vi "gyro-pll-V2.vi"() -> ()   [LabVIEW 2017]
uses:
  lorentzian.ctl
  circle corners.ctl
  pid -- parameters.ctl
  <vilib>/event_ctls.llb/eventvkey.ctl
  cursor winow.ctl
  show-win- control.ctl
  PID action.ctl
  PLL data source.ctl
  cursor window action.ctl
  agregator -- action.ctl
  interpolation state - real.ctl
  data source action.ctl
  four-corner circle transformation.ctl
  cursor action.ctl
  publisher action.ctl
  d67dc248-e042-8a4a-b341-023c3e33f963.vi
  linear interpolation - real.vi
  <vilib>/Array/Sort 2D Array - Pop Stack.vi
  <vilib>/Array/Sort 2D Array - Push Stack.vi
  draw a line.vi
  draw a circle.vi
  linear interpolation iiii- complex.vi
  Q - not nan -- real.vi
  generate linear region.vi
panel:
  in  "all 3":enum32{"all", "other"}(tab)
  in  "reset freq! :r":bool
  in  "dt (sec)":dbl=0.05 format="%#_10f"
  out "Plot: complex plane - filter":cluster{dbl[], dbl[]}[](graph)=[{[1.2813614834440607e-05, 1.2784806307815229e-05, 1.2698431267884004e-05, 1.2554641245817403e-05, 1.235368849817431e-05, 1.2095925564358299e-05, 1.17818046481437e-05, 1.1411876824356577e-05, 1.0986791072102168e-05, 1.0507293136235029e-05, 9.97422421906916e-06, 9.388519504623323e-06, 8.75120651799044e-06, 8.063403322709483e-06, 7.326316559302067e-06, 6.54123932841497e-06, 5.709548922282207e-06, 4.832704408486439e-06, 3.912244070258618e-06, 2.949782707806539e-06, 1.947008805406491e-06, 9.056815692281653e-07, -1.7237215891082665e-07, -1.2852611064461961e-06, -2.431032888001771e-06, -3.6076774305368316e-06, -4.81313049969727e-06, -6.045277321184067e-06, -7.301956290786042e-06, -8.580962766568125e-06, -9.880052936562472e-06, -1.1196947755177101e-05, -1.2529336941416313e-05, -1.3874883031898544e-05, -1.5231225481561452e-05, -1.6595984804860076e-05, -1.7966766750193015e-05, -1.9341166500233316e-05, -2.0716772890795228e-05, -2.209117264083553e-05, -2.3461954586168464e-05, -2.4826713909467085e-05, -2.618305635913e-05, -2.752860244961223e-05, -2.886099163585144e-05, -3.017788645446607e-05, -3.147697662446042e-05, -3.2755983100242503e-05, -3.401266206984447e-05, -3.524480889133127e-05, -3.6450261960491715e-05, -3.762690650302677e-05, -3.877267828458235e-05, -3.9885567232117724e-05, -4.0963620960256705e-05, -4.200494819643504e-05, -4.300772209883508e-05, -4.3970183461287165e-05, -4.4890643799514986e-05, -4.576748831331076e-05, -4.659917871944352e-05, -4.738425595033061e-05, -4.8121342713738026e-05, -4.8809145909018984e-05, -4.9446458895651866e-05, -5.003216361009771e-05, -5.056523252726357e-05, -5.104473046313072e-05, -5.1469816215385134e-05, -5.183974403917225e-05, -5.215386495538684e-05, -5.241162788920287e-05, -5.2612580636845954e-05, -5.275637065891256e-05, -5.2842745698843786e-05, -5.2871554225469164e-05, -5.2842745698843786e-05, -5.275637065891256e-05, -5.2612580636845954e-05, -5.241162788920287e-05, -5.2153864955386856e-05, -5.183974403917226e-05, -5.1469816215385134e-05, -5.104473046313072e-05, -5.0565232527263586e-05, -5.003216361009772e-05, -4.944645889565188e-05, -4.8809145909019e-05, -4.812134271373804e-05, -4.738425595033063e-05, -4.659917871944353e-05, -4.576748831331078e-05, -4.4890643799515e-05, -4.397018346128718e-05, -4.3007722098835096e-05, -4.200494819643505e-05, -4.096362096025673e-05, -3.9885567232117744e-05, -3.8772678284582364e-05, -3.762690650302679e-05, -3.645026196049173e-05, -3.5244808891331293e-05, -3.401266206984449e-05, -3.275598310024252e-05, -3.1476976624460435e-05, -3.0177886454466085e-05, -2.8860991635851447e-05, -2.7528602449612266e-05, -2.6183056359130033e-05, -2.4826713909467122e-05, -2.3461954586168495e-05, -2.209117264083556e-05, -2.0716772890795258e-05, -1.9341166500233336e-05, -1.796676675019304e-05, -1.65959848048601e-05, -1.5231225481561472e-05, -1.387488303189856e-05, -1.2529336941416328e-05, -1.1196947755177116e-05, -9.880052936562479e-06, -8.580962766568159e-06, -7.301956290786074e-06, -6.045277321184099e-06, -4.813130499697297e-06, -3.6076774305368553e-06, -2.431032888001795e-06, -1.2852611064462199e-06, -1.7237215891084359e-07, 9.056815692281483e-07, 1.9470088054064774e-06, 2.949782707806522e-06, 3.912244070258608e-06, 4.832704408486426e-06, 5.7095489222822e-06, 6.541239328414966e-06, 7.3263165593020436e-06, 8.063403322709466e-06, 8.751206517990427e-06, 9.388519504623309e-06, 9.97422421906915e-06, 1.0507293136235015e-05, 1.0986791072102155e-05, 1.1411876824356577e-05, 1.17818046481437e-05, 1.2095925564358292e-05, 1.235368849817431e-05, 1.2554641245817403e-05, 1.2698431267884004e-05, 1.2784806307815229e-05], [3.545285490891632e-05, 3.682815960626468e-05, 3.820105155184222e-05, 3.956912222666456e-05, 4.0929971569894545e-05, 4.2281212189364424e-05, 4.3620473549873006e-05, 4.4945406131909886e-05, 4.625368555351105e-05, 4.754301664801469e-05, 4.881113749056338e-05, 5.0055823366288934e-05, 5.127489067321824e-05, 5.246620075305308e-05, 5.362766364310354e-05, 5.4757241742792726e-05, 5.585295338830057e-05, 5.6912876329075535e-05, 5.7935151100115256e-05, 5.891798428410004e-05, 5.9859651657656206e-05, 6.0758501216229826e-05, 6.161295607226402e-05, 6.24215172215956e-05, 6.31827661732177e-05, 6.389536743779506e-05, 6.455807087056606e-05, 6.516971386452149e-05, 6.572922339001227e-05, 6.623561787720805e-05, 6.668800893810432e-05, 6.708560292505672e-05, 6.742770232310883e-05, 6.771370697367026e-05, 6.794311512739893e-05, 6.811552432443979e-05, 6.823063210047616e-05, 6.8288236517355e-05, 6.8288236517355e-05, 6.823063210047616e-05, 6.811552432443979e-05, 6.794311512739893e-05, 6.771370697367026e-05, 6.742770232310883e-05, 6.708560292505674e-05, 6.668800893810432e-05, 6.623561787720805e-05, 6.572922339001227e-05, 6.516971386452149e-05, 6.455807087056606e-05, 6.389536743779506e-05, 6.31827661732177e-05, 6.242151722159561e-05, 6.161295607226403e-05, 6.075850121622983e-05, 5.985965165765622e-05, 5.8917984284100045e-05, 5.793515110011527e-05, 5.691287632907554e-05, 5.585295338830058e-05, 5.475724174279273e-05, 5.362766364310355e-05, 5.246620075305309e-05, 5.1274890673218255e-05, 5.005582336628895e-05, 4.8811137490563386e-05, 4.7543016648014695e-05, 4.625368555351106e-05, 4.4945406131909906e-05, 4.3620473549873027e-05, 4.228121218936444e-05, 4.092997156989456e-05, 3.9569122226664574e-05, 3.8201051551842225e-05, 3.682815960626469e-05, 3.545285490891634e-05, 3.407755021156798e-05, 3.270465826599045e-05, 3.13365875911681e-05, 2.9975738247938106e-05, 2.8624497628468227e-05, 2.7285236267959645e-05, 2.596030368592278e-05, 2.4652024264321608e-05, 2.336269316981797e-05, 2.209457232726928e-05, 2.0849886451543717e-05, 1.963081914461441e-05, 1.8439509064779572e-05, 1.727804617472912e-05, 1.614846807503993e-05, 1.5052756429532084e-05, 1.3992833488757123e-05, 1.2970558717717392e-05, 1.198772553373261e-05, 1.1046058160176439e-05, 1.0147208601602828e-05, 9.292753745568634e-06, 8.484192596237056e-06, 7.72294364461495e-06, 7.010342380037596e-06, 6.347638947266588e-06, 5.735995953311157e-06, 5.176486427820386e-06, 4.670091940624589e-06, 4.2177008797283295e-06, 3.820106892775922e-06, 3.478007494723825e-06, 3.1920028441623845e-06, 2.9625946904337074e-06, 2.7901854933928613e-06, 2.675077717356487e-06, 2.6174733004776394e-06, 2.6174733004776394e-06, 2.675077717356487e-06, 2.7901854933928545e-06, 2.9625946904337074e-06, 3.1920028441623777e-06, 3.4780074947238183e-06, 3.820106892775915e-06, 4.217700879728323e-06, 4.670091940624575e-06, 5.176486427820369e-06, 5.7359959533111404e-06, 6.347638947266571e-06, 7.010342380037572e-06, 7.722943644614927e-06, 8.484192596237036e-06, 9.292753745568607e-06, 1.0147208601602805e-05, 1.1046058160176422e-05, 1.1987725533732593e-05, 1.2970558717717375e-05, 1.3992833488757099e-05, 1.5052756429532063e-05, 1.6148468075039908e-05, 1.7278046174729072e-05, 1.8439509064779535e-05, 1.9630819144614373e-05, 2.084988645154368e-05, 2.209457232726924e-05, 2.3362693169817932e-05, 2.465202426432157e-05, 2.5960303685922738e-05, 2.7285236267959618e-05, 2.86244976284682e-05, 2.9975738247938083e-05, 3.133658759116807e-05, 3.270465826599042e-05, 3.407755021156795e-05]}, {[-4.107222204249114e-06, -5.699396953375631e-06, -7.291571702502146e-06, -8.883746451628662e-06, -1.0475921200755179e-05, -1.2068095949881695e-05, -1.366027069900821e-05, -1.5252445448134727e-05, -1.6844620197261244e-05, -1.843679494638776e-05, -2.0028969695514277e-05, -2.1621144444640793e-05, -2.3213319193767307e-05, -2.4805493942893823e-05, -2.639766869202034e-05, -2.7989843441146856e-05, -2.9582018190273373e-05, -3.1174192939399886e-05, -3.2766367688526406e-05, -3.4358542437652926e-05], [6.727721046188663e-06, 9.60023443246143e-06, 1.2472747818734195e-05, 1.534526120500696e-05, 1.8217774591279727e-05, 2.1090287977552493e-05, 2.396280136382526e-05, 2.6835314750098024e-05, 2.970782813637079e-05, 3.2580341522643556e-05, 3.545285490891632e-05, 3.832536829518909e-05, 4.1197881681461854e-05, 4.407039506773462e-05, 4.6942908454007386e-05, 4.981542184028015e-05, 5.268793522655292e-05, 5.556044861282568e-05, 5.843296199909845e-05, 6.130547538537121e-05]}, {[-4.875410355824193e-05, -4.5881590171969166e-05, -4.30090767856964e-05, -4.0136563399423635e-05, -3.726405001315087e-05, -3.43915366268781e-05, -3.1519023240605344e-05, -2.8646509854332574e-05, -2.577399646805981e-05, -2.2901483081787043e-05, -2.0028969695514277e-05, -1.7156456309241514e-05, -1.4283942922968748e-05, -1.1411429536695983e-05, -8.538916150423217e-06, -5.666402764150451e-06, -2.793889377877685e-06, 7.862400839508097e-08, 2.951137394667847e-06, 5.823650780940613e-06], [1.953110741765116e-05, 2.1123282166777676e-05, 2.2715456915904193e-05, 2.430763166503071e-05, 2.5899806414157222e-05, 2.7491981163283742e-05, 2.9084155912410256e-05, 3.067633066153677e-05, 3.226850541066329e-05, 3.386068015978981e-05, 3.545285490891632e-05, 3.7045029658042835e-05, 3.863720440716935e-05, 4.022937915629587e-05, 4.182155390542239e-05, 4.34137286545489e-05, 4.5005903403675415e-05, 4.6598078152801935e-05, 4.8190252901928455e-05, 4.978242765105497e-05]}, {[-6.155748992970442e-05, -5.581246315715889e-05, -5.006743638461336e-05, -4.432240961206783e-05, -3.85773828395223e-05, -3.2832356066976766e-05, -2.7087329294431234e-05, -2.1342302521885702e-05, -1.559727574934017e-05, -9.852248976794639e-06, -4.107222204249107e-06, 1.6378045682964245e-06, 7.382831340841956e-06, 1.3127858113387488e-05, 1.887288488593302e-05, 2.461791165847855e-05, 3.0362938431024083e-05, 3.6107965203569615e-05, 4.185299197611515e-05, 4.759801874866068e-05], [-2.5115773936341655e-05, -2.1931424438088622e-05, -1.874707493983559e-05, -1.556272544158256e-05, -1.2378375943329526e-05, -9.194026445076493e-06, -6.009676946823463e-06, -2.8253274485704296e-06, 3.5902204968260365e-07, 3.543371547935637e-06, 6.72772104618867e-06, 9.912070544441703e-06, 1.309642004269473e-05, 1.6280769540947763e-05, 1.9465119039200796e-05, 2.264946853745383e-05, 2.5833818035706863e-05, 2.9018167533959896e-05, 3.220251703221293e-05, 3.538686653046596e-05]}]
  in  "PID parameters :{}[]":T1={"I (sec)"=1.05568883726763, "P (sec)"=1.0091249923988408} {"P (sec)" scale=0.01..10.0; "I (sec)" scale=0.01..10.0}
  in  "visc hist time (sec)":dbl=5.0 format="%#_10f"
  in  "circle lorentzian":T2={"Amplitude (V)"=0.0014148170690314607, "omega0 (Hz)"=45421.57991847975, "Gamma (Hz)"=43.078737233394115, "phase (rad)"=3.647715388411055, "Q"=1054.3851290810235, "Norm  Ampl"=nan, "z (inf)"=-4.107222204249114e-06+6.727721046188663e-06i, "4corners"={"z (-pi/2)"=-4.875410355824193e-05+1.9531107417651163e-05i, "z(inf)"=-4.107222204249114e-06+6.727721046188663e-06i, "z (pi/2)"=8.696164167213385e-06+5.137460240018148e-05i, "z center"=-2.0028969695514273e-05+3.545285490891632e-05i, "z(0)"=-3.595071718677943e-05+6.417798877164398e-05i, "radius"=3.2842584529954884e-05}} {"z (inf)" format="%#9_9f"; "Q" format="%#9_9f"; "phase (rad)" format="%#9_9f"; "Gamma (Hz)" format="%#9_9f"; "omega0 (Hz)" format="%#9_9f"}
  in  "time int ave time (sec)":dbl=0.05 format="%#_10f"
  in  "get fit! :q":bool
  in  "PLL away! :@":bool
  out "zi freq (Hz)":dbl=45590.53325451146 format="%#.4f"
  out "delta freq (Hz)":dbl=168.9533360317073 format="%#.8f"
  in  "PLL limits (Hz)":dbl=5000.0 format="%#.2f"
  in  "PLL data source":T4=enum."MFLI"
  in  "cursor bracket: fit boundaries":T5={"left"=20223.692861806387, "right "=24717.846831096696, "center"=22470.76984645154, "window"=4494.153969290309, "cursors"=[0, 1, 2], "relative"=0, "absolute"=0, "fixed vertical offset"=0.0, "vertical offset"=0.0, "skew"=0.0, "default window frac"=0.1, "kind"=enum."symmetric", "skew.left"=0.5, "skew.right"=0.5, "Plot ref"=refnum, "wing order"=enum."forw"}
  out "VKey":T6
  out "Char":i16=122
  in  "lorentzian -- basic":T2={"Amplitude (V)"=1.0, "omega0 (Hz)"=1000.0, "Gamma (Hz)"=3.0, "phase (rad)"=0.0, "Q"=300.0, "Norm  Ampl"=nan, "z (inf)"=0.0+0.0i, "4corners"={"z (-pi/2)"=9.277908004825974e-07+0.0007240755403629966i, "z(inf)"=2.6527949823343002e-05+0.0007477540585896028i, "z (pi/2)"=2.8494315967368497e-06+0.0007733542176124632i, "z center"=1.8886111986097237e-06+0.0007487148789877299i, "z(0)"=-2.2750727426123552e-05+0.000749675699385857i, "radius"=2.4658065287076567e-05}} {"z (inf)" format="%#9_9f"; "Q" format="%#9_9f"; "phase (rad)" format="%#9_9f"; "Gamma (Hz)" format="%#9_9f"; "omega0 (Hz)" format="%#9_9f"}
  out "DO reset freq !":bool
  in  "save lor for later":bool
  in  "reset lorentzian from basic":bool
  in  "Do reset frequency source":dbl=15.0 format="%#_10f"
  in  "Do reset frequency -- PID action":T7=enum."reset frequency"
  in  "all":enum32{"all", "other"}(tab)
  in  "reset win from freq !":bool
  in  "reset freq from win !":bool
  in  "send for fit!":bool
  out "Plot: complex- hist":cluster{dbl[], dbl[]}[](graph)=[{[-1.281770488197954e-05, -1.0986465994251437e-05, -6.882277068596139e-06, -1.0956775876071293e-05, -6.698135551181071e-06, -4.290132536004875e-06, -9.884114205234754e-06, -1.0020825799021037e-05, -1.0594885594792778e-05, -1.1315291508425677e-05, -9.15588407390866e-06, -4.631085114607762e-06, -9.91714593188108e-06, -1.1229612675301296e-05, -3.7616560713859013e-06, -8.359687227641351e-06, -1.2250832382384907e-05, -7.790134627243845e-06, -9.342526339103081e-06, -1.4326621095772142e-05, -1.5233280532867308e-05, -8.680230516053846e-06, -1.0092209301965068e-05, -1.1126455180992973e-05, -1.450326589164611e-05, -5.246423985745027e-06, -3.6636994414210996e-06, -5.141838176586089e-06, -1.0012731994795598e-05, -1.5335458675967136e-05, -1.5049525631563538e-05, -1.6069153025824554e-05, -8.141448343003425e-06, -7.412163963946879e-06, -1.2430596668377613e-05, -1.3231583279096937e-05, -6.985101526890639e-06, -6.490446532337178e-06, -9.373512369438486e-06, -1.2126573717328789e-05, -1.589980051855066e-05, -1.1354584338626872e-05, -8.824369474721001e-06, -9.99549965874622e-07, -6.288455267304482e-06, -7.484835846038533e-06, -1.351758082676016e-05, -9.828075336477092e-06, -1.1524401297069373e-05, -1.587464391008797e-05, -1.0557451032928354e-05, -1.3139806431129755e-05, -1.2011711561005575e-05, -1.1843224223572645e-05, -1.37278337116776e-05, -1.6522056027489975e-05, -1.2383234897091292e-05, -8.10061086687687e-06, -5.225988471535249e-06, -3.4747132306206463e-06, -9.256075255275086e-06, -1.113538910524981e-05, -1.0058288945367669e-05, -1.0233727177421544e-05, -8.648566858261817e-06, -8.711623226434552e-06, -1.1066342002860999e-05, -1.1269186189822962e-05, -9.535872752272664e-06, -7.947195421785513e-06, -2.452968790242578e-06, -8.09754757022516e-06, -6.77439165155316e-06, -1.3610673819421092e-05, -1.1234462535209906e-05, -8.525491417347455e-06, -1.392286151503345e-05, -6.713947219797658e-06, -6.725420448067176e-06, -6.755292683180116e-06, -8.367269690585905e-06, -1.0878166562867951e-05, -1.4503510879987953e-05, -1.248913934388176e-05, -9.905257659579364e-06, -1.0500128831114514e-05, -1.212190723888663e-05, -1.0435993159380175e-05, -4.5051603662442005e-06, -9.992924080682386e-06, -5.240584718574565e-06, -7.197456861593793e-06, -9.92233566832843e-06, -7.377046557639752e-06, -8.116089144205894e-06, -7.294297372002839e-06, -2.9009344623999418e-06, -7.1961787793630815e-06, -6.897321683140279e-06, -1.3261197639667919e-05], [5.706075424171509e-06, -1.1630478027538063e-06, -3.525889919298938e-06, -1.7232249579361585e-06, 3.037512629820769e-06, 5.382037422375056e-06, 7.061626647765622e-06, 1.015592289042986e-05, 6.011991857808628e-06, 9.202991740167639e-06, 8.434441080095082e-06, 6.850955786302219e-06, 1.2665083395419556e-05, 9.806056240748531e-06, 6.1280478362699535e-06, 7.380703233698666e-06, 4.597579229991622e-06, 3.273804316073506e-06, 6.20732814113902e-06, 1.500419119676377e-06, 3.6290960078291793e-06, 3.1569128782905418e-06, 7.704539470117948e-06, 1.1767566699238926e-05, 1.6401704723257656e-05, 1.773510518306169e-05, 1.2043904088923593e-05, 1.0448690498379654e-05, 5.320948138670971e-06, 7.029982849173579e-06, 7.638521311216531e-06, 1.334940401664198e-05, 1.1916412029374287e-05, 8.520753444581032e-06, 1.041158118661469e-05, 3.5441337799059673e-06, 5.204323559640508e-06, 2.871329995299419e-06, 5.626692421104822e-06, 1.2367157694471746e-05, 6.94819555815912e-06, 7.5136952860385745e-06, 5.595164995738646e-06, -8.017660632431858e-08, 4.884120262176944e-06, 1.3265296378628144e-05, 1.0419894845070167e-05, 7.067744798801493e-06, 3.381769007333527e-06, 5.722049434823149e-06, 5.425078715713811e-06, 6.195883948970877e-06, 8.230847301668298e-06, 8.317429156341073e-06, 1.0934201336945204e-05, 6.657226105024734e-06, 3.136753688770917e-06, 7.125990080076144e-06, 1.0622469258830631e-05, 6.566659415766181e-06, 1.338506083085556e-05, 6.687905142718035e-06, 6.291463087058234e-06, 9.921191747097013e-06, 1.0284209077115023e-05, 1.0653382843430736e-05, 1.6941958741224393e-05, 1.2704846367190809e-05, 1.393377923968955e-05, 9.477494020546201e-06, 1.029700437532171e-05, 9.78797003738044e-06, -4.1512948456535147e-07, 3.4799239643482737e-06, 1.017011873794103e-05, 1.0556332185592857e-05, 8.426406058619873e-06, 1.2298688026322897e-05, 6.880312085661992e-06, 5.67266378946385e-06, 9.975259828108888e-06, 7.693594636268902e-06, 8.049333768204717e-06, 5.9931496138540715e-06, 7.859370548593827e-06, 6.540359452101423e-06, 7.503472627360372e-06, 1.3451819121305734e-05, 1.2886720756408641e-05, 9.644031995046428e-06, 6.8135854145748034e-06, 4.454962679522251e-06, 1.042299277790087e-05, 9.437539068479638e-06, 6.283286552223761e-06, 5.563695576337742e-06, 6.333150901852445e-06, 6.151665278453125e-06, 7.035160108888859e-06, 1.110513348159719e-05]}]
  out "Plot: hist":cluster{"all rows":dbl[], "all rows":dbl[]}[](graph)=[{"all rows"=[45590.53325451146, 45590.53325451146, 45590.53325451146, 45590.53325451146, 45590.53325451146, 45590.53325451146, 45590.53325451146, 45590.53325451146, 45590.53325451146, 45590.53325451146, 45590.53325451146, 45590.53325451146, 45590.53325451146, 45590.53325451146, 45590.53325451146, 45590.53325451146, 45590.53325451146, 45590.53325451146, 45590.53325451146, 45590.53325451146, 45590.53325451146, 45590.53325451146, 45590.53325451146, 45590.53325451146, 45590.53325451146, 45590.53325451146, 45590.53325451146, 45590.53325451146, 45590.53325451146, 45590.53325451146, 45590.53325451146, 45590.53325451146, 45590.53325451146, 45590.53325451146, 45590.53325451146, 45590.53325451146, 45590.53325451146, 45590.53325451146, 45590.53325451146, 45590.53325451146, 45590.53325451146, 45590.53325451146, 45590.53325451146, 45590.53325451146, 45590.53325451146, 45590.53325451146, 45590.53325451146, 45590.53325451146, 45590.53325451146, 45590.53325451146, 45590.53325451146, 45590.53325451146, 45590.53325451146, 45590.53325451146, 45590.53325451146, 45590.53325451146, 45590.53325451146, 45590.53325451146, 45590.53325451146, 45590.53325451146, 45590.53325451146, 45590.53325451146, 45590.53325451146, 45590.53325451146, 45590.53325451146, 45590.53325451146, 45590.53325451146, 45590.53325451146, 45590.53325451146, 45590.53325451146, 45590.53325451146, 45590.53325451146, 45590.53325451146, 45590.53325451146, 45590.53325451146, 45590.53325451146, 45590.53325451146, 45590.53325451146, 45590.53325451146, 45590.53325451146, 45590.53325451146, 45590.53325451146, 45590.53325451146, 45590.53325451146, 45590.53325451146, 45590.53325451146, 45590.53325451146, 45590.53325451146, 45590.53325451146, 45590.53325451146, 45590.53325451146, 45590.53325451146, 45590.53325451146, 45590.53325451146, 45590.53325451146, 45590.53325451146, 45590.53325451146, 45590.53325451146, 45590.53325451146, 45590.53325451146], "all rows"=[-1.281770488197954e-05, -1.0986465994251437e-05, -6.882277068596139e-06, -1.0956775876071293e-05, -6.698135551181071e-06, -4.290132536004875e-06, -9.884114205234754e-06, -1.0020825799021037e-05, -1.0594885594792778e-05, -1.1315291508425677e-05, -9.15588407390866e-06, -4.631085114607762e-06, -9.91714593188108e-06, -1.1229612675301296e-05, -3.7616560713859013e-06, -8.359687227641351e-06, -1.2250832382384907e-05, -7.790134627243845e-06, -9.342526339103081e-06, -1.4326621095772142e-05, -1.5233280532867308e-05, -8.680230516053846e-06, -1.0092209301965068e-05, -1.1126455180992973e-05, -1.450326589164611e-05, -5.246423985745027e-06, -3.6636994414210996e-06, -5.141838176586089e-06, -1.0012731994795598e-05, -1.5335458675967136e-05, -1.5049525631563538e-05, -1.6069153025824554e-05, -8.141448343003425e-06, -7.412163963946879e-06, -1.2430596668377613e-05, -1.3231583279096937e-05, -6.985101526890639e-06, -6.490446532337178e-06, -9.373512369438486e-06, -1.2126573717328789e-05, -1.589980051855066e-05, -1.1354584338626872e-05, -8.824369474721001e-06, -9.99549965874622e-07, -6.288455267304482e-06, -7.484835846038533e-06, -1.351758082676016e-05, -9.828075336477092e-06, -1.1524401297069373e-05, -1.587464391008797e-05, -1.0557451032928354e-05, -1.3139806431129755e-05, -1.2011711561005575e-05, -1.1843224223572645e-05, -1.37278337116776e-05, -1.6522056027489975e-05, -1.2383234897091292e-05, -8.10061086687687e-06, -5.225988471535249e-06, -3.4747132306206463e-06, -9.256075255275086e-06, -1.113538910524981e-05, -1.0058288945367669e-05, -1.0233727177421544e-05, -8.648566858261817e-06, -8.711623226434552e-06, -1.1066342002860999e-05, -1.1269186189822962e-05, -9.535872752272664e-06, -7.947195421785513e-06, -2.452968790242578e-06, -8.09754757022516e-06, -6.77439165155316e-06, -1.3610673819421092e-05, -1.1234462535209906e-05, -8.525491417347455e-06, -1.392286151503345e-05, -6.713947219797658e-06, -6.725420448067176e-06, -6.755292683180116e-06, -8.367269690585905e-06, -1.0878166562867951e-05, -1.4503510879987953e-05, -1.248913934388176e-05, -9.905257659579364e-06, -1.0500128831114514e-05, -1.212190723888663e-05, -1.0435993159380175e-05, -4.5051603662442005e-06, -9.992924080682386e-06, -5.240584718574565e-06, -7.197456861593793e-06, -9.92233566832843e-06, -7.377046557639752e-06, -8.116089144205894e-06, -7.294297372002839e-06, -2.9009344623999418e-06, -7.1961787793630815e-06, -6.897321683140279e-06, -1.3261197639667919e-05]}, {"all rows"=[45590.53325451146, 45590.53325451146, 45590.53325451146, 45590.53325451146, 45590.53325451146, 45590.53325451146, 45590.53325451146, 45590.53325451146, 45590.53325451146, 45590.53325451146, 45590.53325451146, 45590.53325451146, 45590.53325451146, 45590.53325451146, 45590.53325451146, 45590.53325451146, 45590.53325451146, 45590.53325451146, 45590.53325451146, 45590.53325451146, 45590.53325451146, 45590.53325451146, 45590.53325451146, 45590.53325451146, 45590.53325451146, 45590.53325451146, 45590.53325451146, 45590.53325451146, 45590.53325451146, 45590.53325451146, 45590.53325451146, 45590.53325451146, 45590.53325451146, 45590.53325451146, 45590.53325451146, 45590.53325451146, 45590.53325451146, 45590.53325451146, 45590.53325451146, 45590.53325451146, 45590.53325451146, 45590.53325451146, 45590.53325451146, 45590.53325451146, 45590.53325451146, 45590.53325451146, 45590.53325451146, 45590.53325451146, 45590.53325451146, 45590.53325451146, 45590.53325451146, 45590.53325451146, 45590.53325451146, 45590.53325451146, 45590.53325451146, 45590.53325451146, 45590.53325451146, 45590.53325451146, 45590.53325451146, 45590.53325451146, 45590.53325451146, 45590.53325451146, 45590.53325451146, 45590.53325451146, 45590.53325451146, 45590.53325451146, 45590.53325451146, 45590.53325451146, 45590.53325451146, 45590.53325451146, 45590.53325451146, 45590.53325451146, 45590.53325451146, 45590.53325451146, 45590.53325451146, 45590.53325451146, 45590.53325451146, 45590.53325451146, 45590.53325451146, 45590.53325451146, 45590.53325451146, 45590.53325451146, 45590.53325451146, 45590.53325451146, 45590.53325451146, 45590.53325451146, 45590.53325451146, 45590.53325451146, 45590.53325451146, 45590.53325451146, 45590.53325451146, 45590.53325451146, 45590.53325451146, 45590.53325451146, 45590.53325451146, 45590.53325451146, 45590.53325451146, 45590.53325451146, 45590.53325451146, 45590.53325451146], "all rows"=[5.706075424171509e-06, -1.1630478027538063e-06, -3.525889919298938e-06, -1.7232249579361585e-06, 3.037512629820769e-06, 5.382037422375056e-06, 7.061626647765622e-06, 1.015592289042986e-05, 6.011991857808628e-06, 9.202991740167639e-06, 8.434441080095082e-06, 6.850955786302219e-06, 1.2665083395419556e-05, 9.806056240748531e-06, 6.1280478362699535e-06, 7.380703233698666e-06, 4.597579229991622e-06, 3.273804316073506e-06, 6.20732814113902e-06, 1.500419119676377e-06, 3.6290960078291793e-06, 3.1569128782905418e-06, 7.704539470117948e-06, 1.1767566699238926e-05, 1.6401704723257656e-05, 1.773510518306169e-05, 1.2043904088923593e-05, 1.0448690498379654e-05, 5.320948138670971e-06, 7.029982849173579e-06, 7.638521311216531e-06, 1.334940401664198e-05, 1.1916412029374287e-05, 8.520753444581032e-06, 1.041158118661469e-05, 3.5441337799059673e-06, 5.204323559640508e-06, 2.871329995299419e-06, 5.626692421104822e-06, 1.2367157694471746e-05, 6.94819555815912e-06, 7.5136952860385745e-06, 5.595164995738646e-06, -8.017660632431858e-08, 4.884120262176944e-06, 1.3265296378628144e-05, 1.0419894845070167e-05, 7.067744798801493e-06, 3.381769007333527e-06, 5.722049434823149e-06, 5.425078715713811e-06, 6.195883948970877e-06, 8.230847301668298e-06, 8.317429156341073e-06, 1.0934201336945204e-05, 6.657226105024734e-06, 3.136753688770917e-06, 7.125990080076144e-06, 1.0622469258830631e-05, 6.566659415766181e-06, 1.338506083085556e-05, 6.687905142718035e-06, 6.291463087058234e-06, 9.921191747097013e-06, 1.0284209077115023e-05, 1.0653382843430736e-05, 1.6941958741224393e-05, 1.2704846367190809e-05, 1.393377923968955e-05, 9.477494020546201e-06, 1.029700437532171e-05, 9.78797003738044e-06, -4.1512948456535147e-07, 3.4799239643482737e-06, 1.017011873794103e-05, 1.0556332185592857e-05, 8.426406058619873e-06, 1.2298688026322897e-05, 6.880312085661992e-06, 5.67266378946385e-06, 9.975259828108888e-06, 7.693594636268902e-06, 8.049333768204717e-06, 5.9931496138540715e-06, 7.859370548593827e-06, 6.540359452101423e-06, 7.503472627360372e-06, 1.3451819121305734e-05, 1.2886720756408641e-05, 9.644031995046428e-06, 6.8135854145748034e-06, 4.454962679522251e-06, 1.042299277790087e-05, 9.437539068479638e-06, 6.283286552223761e-06, 5.563695576337742e-06, 6.333150901852445e-06, 6.151665278453125e-06, 7.035160108888859e-06, 1.110513348159719e-05]}]
  out "window":T8={"cen (Hz)"=32820.887133413584, "win (Hz)"=623.378672999308, "left (Hz)"=32509.19779691393, "right (Hz)"=33132.57646991324}
  out "freq out":dbl[](array[numeric])=[45590.53325451146, 45590.53325451146, 45590.53325451146, 45590.53325451146, 45590.53325451146, 45590.53325451146, 45590.53325451146, 45590.53325451146, 45590.53325451146, 45590.53325451146, 45590.53325451146, 45590.53325451146, 45590.53325451146, 45590.53325451146, 45590.53325451146, 45590.53325451146, 45590.53325451146, 45590.53325451146, 45590.53325451146, 45590.53325451146, 45590.53325451146, 45590.53325451146, 45590.53325451146, 45590.53325451146, 45590.53325451146, 45590.53325451146, 45590.53325451146, 45590.53325451146, 45590.53325451146, 45590.53325451146, 45590.53325451146, 45590.53325451146, 45590.53325451146, 45590.53325451146, 45590.53325451146, 45590.53325451146, 45590.53325451146, 45590.53325451146, 45590.53325451146, 45590.53325451146, 45590.53325451146, 45590.53325451146, 45590.53325451146, 45590.53325451146, 45590.53325451146, 45590.53325451146, 45590.53325451146, 45590.53325451146, 45590.53325451146, 45590.53325451146, 45590.53325451146, 45590.53325451146, 45590.53325451146, 45590.53325451146, 45590.53325451146, 45590.53325451146, 45590.53325451146, 45590.53325451146, 45590.53325451146, 45590.53325451146, 45590.53325451146, 45590.53325451146, 45590.53325451146, 45590.53325451146, 45590.53325451146, 45590.53325451146, 45590.53325451146, 45590.53325451146, 45590.53325451146, 45590.53325451146, 45590.53325451146, 45590.53325451146, 45590.53325451146, 45590.53325451146, 45590.53325451146, 45590.53325451146, 45590.53325451146, 45590.53325451146, 45590.53325451146, 45590.53325451146, 45590.53325451146, 45590.53325451146, 45590.53325451146, 45590.53325451146, 45590.53325451146, 45590.53325451146, 45590.53325451146, 45590.53325451146, 45590.53325451146, 45590.53325451146, 45590.53325451146, 45590.53325451146, 45590.53325451146, 45590.53325451146, 45590.53325451146, 45590.53325451146, 45590.53325451146, 45590.53325451146, 45590.53325451146, 45590.53325451146]
  out "v out":cdb[](array[numeric])=[-1.281770488197954e-05+5.706075424171509e-06i, -1.0986465994251437e-05-1.1630478027538063e-06i, -6.882277068596139e-06-3.525889919298938e-06i, -1.0956775876071293e-05-1.7232249579361585e-06i, -6.698135551181071e-06+3.037512629820769e-06i, -4.290132536004875e-06+5.382037422375056e-06i, -9.884114205234754e-06+7.061626647765622e-06i, -1.0020825799021037e-05+1.015592289042986e-05i, -1.0594885594792778e-05+6.011991857808628e-06i, -1.1315291508425677e-05+9.202991740167639e-06i, -9.15588407390866e-06+8.434441080095082e-06i, -4.631085114607762e-06+6.850955786302219e-06i, -9.91714593188108e-06+1.2665083395419556e-05i, -1.1229612675301296e-05+9.806056240748531e-06i, -3.7616560713859013e-06+6.1280478362699535e-06i, -8.359687227641351e-06+7.380703233698666e-06i, -1.2250832382384907e-05+4.597579229991622e-06i, -7.790134627243845e-06+3.273804316073506e-06i, -9.342526339103081e-06+6.20732814113902e-06i, -1.4326621095772142e-05+1.500419119676377e-06i, -1.5233280532867308e-05+3.6290960078291793e-06i, -8.680230516053846e-06+3.1569128782905418e-06i, -1.0092209301965068e-05+7.704539470117948e-06i, -1.1126455180992973e-05+1.1767566699238926e-05i, -1.450326589164611e-05+1.6401704723257656e-05i, -5.246423985745027e-06+1.773510518306169e-05i, -3.6636994414210996e-06+1.2043904088923593e-05i, -5.141838176586089e-06+1.0448690498379654e-05i, -1.0012731994795598e-05+5.320948138670971e-06i, -1.5335458675967136e-05+7.029982849173579e-06i, -1.5049525631563538e-05+7.638521311216531e-06i, -1.6069153025824554e-05+1.334940401664198e-05i, -8.141448343003425e-06+1.1916412029374287e-05i, -7.412163963946879e-06+8.520753444581032e-06i, -1.2430596668377613e-05+1.041158118661469e-05i, -1.3231583279096937e-05+3.5441337799059673e-06i, -6.985101526890639e-06+5.204323559640508e-06i, -6.490446532337178e-06+2.871329995299419e-06i, -9.373512369438486e-06+5.626692421104822e-06i, -1.2126573717328789e-05+1.2367157694471746e-05i, -1.589980051855066e-05+6.94819555815912e-06i, -1.1354584338626872e-05+7.5136952860385745e-06i, -8.824369474721001e-06+5.595164995738646e-06i, -9.99549965874622e-07-8.017660632431858e-08i, -6.288455267304482e-06+4.884120262176944e-06i, -7.484835846038533e-06+1.3265296378628144e-05i, -1.351758082676016e-05+1.0419894845070167e-05i, -9.828075336477092e-06+7.067744798801493e-06i, -1.1524401297069373e-05+3.381769007333527e-06i, -1.587464391008797e-05+5.722049434823149e-06i, -1.0557451032928354e-05+5.425078715713811e-06i, -1.3139806431129755e-05+6.195883948970877e-06i, -1.2011711561005575e-05+8.230847301668298e-06i, -1.1843224223572645e-05+8.317429156341073e-06i, -1.37278337116776e-05+1.0934201336945204e-05i, -1.6522056027489975e-05+6.657226105024734e-06i, -1.2383234897091292e-05+3.136753688770917e-06i, -8.10061086687687e-06+7.125990080076144e-06i, -5.225988471535249e-06+1.0622469258830631e-05i, -3.4747132306206463e-06+6.566659415766181e-06i, -9.256075255275086e-06+1.338506083085556e-05i, -1.113538910524981e-05+6.687905142718035e-06i, -1.0058288945367669e-05+6.291463087058234e-06i, -1.0233727177421544e-05+9.921191747097013e-06i, -8.648566858261817e-06+1.0284209077115023e-05i, -8.711623226434552e-06+1.0653382843430736e-05i, -1.1066342002860999e-05+1.6941958741224393e-05i, -1.1269186189822962e-05+1.2704846367190809e-05i, -9.535872752272664e-06+1.393377923968955e-05i, -7.947195421785513e-06+9.477494020546201e-06i, -2.452968790242578e-06+1.029700437532171e-05i, -8.09754757022516e-06+9.78797003738044e-06i, -6.77439165155316e-06-4.1512948456535147e-07i, -1.3610673819421092e-05+3.4799239643482737e-06i, -1.1234462535209906e-05+1.017011873794103e-05i, -8.525491417347455e-06+1.0556332185592857e-05i, -1.392286151503345e-05+8.426406058619873e-06i, -6.713947219797658e-06+1.2298688026322897e-05i, -6.725420448067176e-06+6.880312085661992e-06i, -6.755292683180116e-06+5.67266378946385e-06i, -8.367269690585905e-06+9.975259828108888e-06i, -1.0878166562867951e-05+7.693594636268902e-06i, -1.4503510879987953e-05+8.049333768204717e-06i, -1.248913934388176e-05+5.9931496138540715e-06i, -9.905257659579364e-06+7.859370548593827e-06i, -1.0500128831114514e-05+6.540359452101423e-06i, -1.212190723888663e-05+7.503472627360372e-06i, -1.0435993159380175e-05+1.3451819121305734e-05i, -4.5051603662442005e-06+1.2886720756408641e-05i, -9.992924080682386e-06+9.644031995046428e-06i, -5.240584718574565e-06+6.8135854145748034e-06i, -7.197456861593793e-06+4.454962679522251e-06i, -9.92233566832843e-06+1.042299277790087e-05i, -7.377046557639752e-06+9.437539068479638e-06i, -8.116089144205894e-06+6.283286552223761e-06i, -7.294297372002839e-06+5.563695576337742e-06i, -2.9009344623999418e-06+6.333150901852445e-06i, -7.1961787793630815e-06+6.151665278453125e-06i, -6.897321683140279e-06+7.035160108888859e-06i, -1.3261197639667919e-05+1.110513348159719e-05i]
  out "zi freq temporary":dbl=45421.57991847975 format="%#.2f"
  out "dev freq":dbl=45421.57991847975 format="%#.2f"
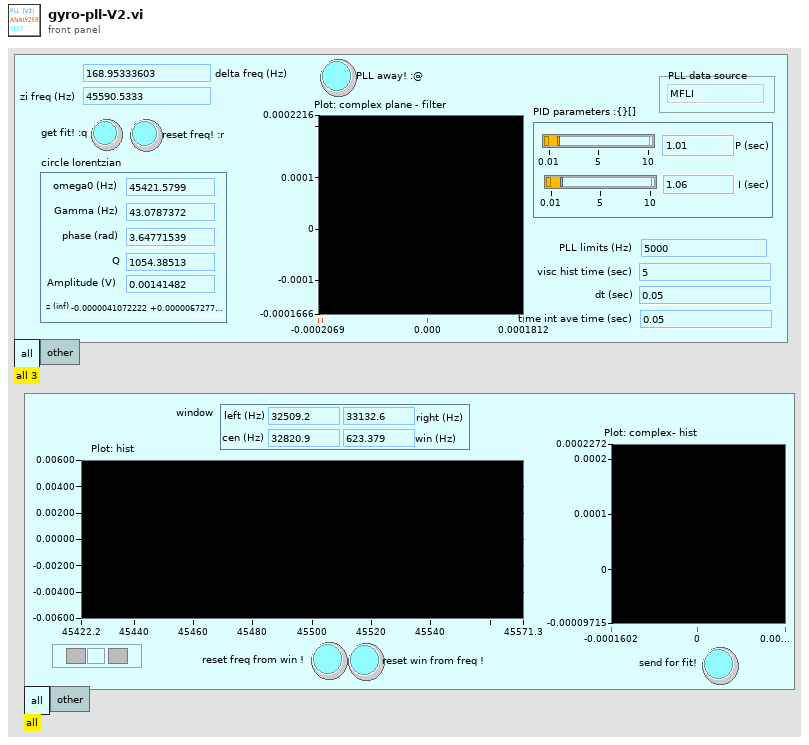
[diagram p1: front panel]
types:
  T1 = typedef "pid -- parameters.ctl" = cluster{"I (sec)":dbl, "P (sec)":dbl}
  T2 = typedef "lorentzian.ctl" = cluster{"Amplitude (V)":dbl, "omega0 (Hz)":dbl, "Gamma (Hz)":dbl, "phase (rad)":dbl, "Q":dbl, "Norm  Ampl":dbl, "z (inf)":cdb, "4corners":T3}
  T3 = typedef "circle corners.ctl" = cluster{"z (-pi/2)":cdb, "z(inf)":cdb, "z (pi/2)":cdb, "z center":cdb, "z(0)":cdb, "radius":dbl}
  T4 = typedef "PLL data source.ctl" = enum16{"meta", "MFLI"}
  T5 = typedef "cursor winow.ctl" = cluster{"left":dbl, "right ":dbl, "center":dbl, "window":dbl, "cursors":i32[], "relative":i32, "absolute":i32, "fixed vertical offset":dbl, "vertical offset":dbl, "skew":dbl, "default window frac":dbl, "kind":enum16{"symmetric", "skewed", "fancy"}, "skew.left":dbl, "skew.right":dbl, "Plot ref":refnum<vi>, "wing order":enum16{"forw", "back"}}
  T6 = typedef "eventvkey.ctl" = enum16{"ASCII", "Enter", "Return", "Shift", "Ctrl", "Alt", "Cmd", "Opt", "Caps", "NumLock", "Clear", "Break", "Up", "Down", "Left", "Right", "Insert", "Delete", "Home", "End", "PageUp", "PageDown", "Escape", "Help", "Pause", "ScrollLock", "F1", "F2", "F3", "F4", "F5", "F6", "F7", "F8", "F9", "F10", "F11", "F12", "F13", "F14", "F15", "F16", "F17", "F18", "F19", "F20", "F21", "F22", "F23", "F24", "Play", "VolumeUp", "VolumeDown", "Mute", "Two Byte Char"}
  T7 = typedef "PID action.ctl" = enum16{"append", "empty!", "reset frequency", "reset from num"}
  T8 = typedef "show-win- control.ctl" = cluster{"cen (Hz)":dbl, "win (Hz)":dbl, "left (Hz)":dbl, "right (Hz)":dbl}
  T9 = typedef "data source action.ctl" = enum16{"set", "get", "init"}
  T10 = typedef "interpolation state - real.ctl" = cluster{"requested size":i32, "Array":dbl[], "actual number of elements":i32}
  T11 = typedef "agregator -- action.ctl" = enum16{"append", "interpolate", "empty!", "force", "init", "scale", "read last"}
  T12 = typedef "cursor window action.ctl" = enum16{"balance", "h. offset change", "cursor moves", "change center", "change window", "init", "check", "reset", "set y to middle", "idle", "-write all Y", "-write left.X", "-write center.X", "-write right.X", "-write all X", "-change center", "-change window", "-change skew", "-read cursor 2", "-read cursor 1", "-read cursor 0", "-read all cursors", "-reset", "-read plot scale", "-set y to middle", "-Q: center.Y is visible", "-Q: window is visible", "-parse center.Y", "-right left from center", "-left move", "-right move", "-set center.Y", "-empty", "-set cursors to default", "-check", "-write center.Y", "-copy cursor 1", "-copy cursor 0", "-copy cursor 2", "move right", "move left", "shrink", "broaden", "skew up", "skew down", "-write plot scale", "zoom X", "change cen&win", "zoom to all data", "color--red", "color--green", "color--yellow", "read", "zoom out", "zoom in", "slide right", "slide left", "set range aspect ratio to 1"}
  T13 = typedef "publisher action.ctl" = enum16{"set", "get"}
  T14 = typedef "cursor action.ctl" = enum16{"range", "read", "write", "check", "zoom out", "smart zoom out", "zoom to aspect ratio 1", "zoom to win", "zoom out 20%", "zoom in 20%"}
  T15 = typedef "four-corner circle transformation.ctl" = enum16{"z(c) z(inf)", "z(c) z(zero)", "fix phase", "calculate lorentzian", "z(0) z(+-pi/2)", "shift to zcenter", "to  canonical", "get canonical phase", "get4corners"}
  T16 = typedef "interpolation state - complex.ctl" = cluster{"requested size":i32, "Array":cdb[], "actual number of elements":i32}
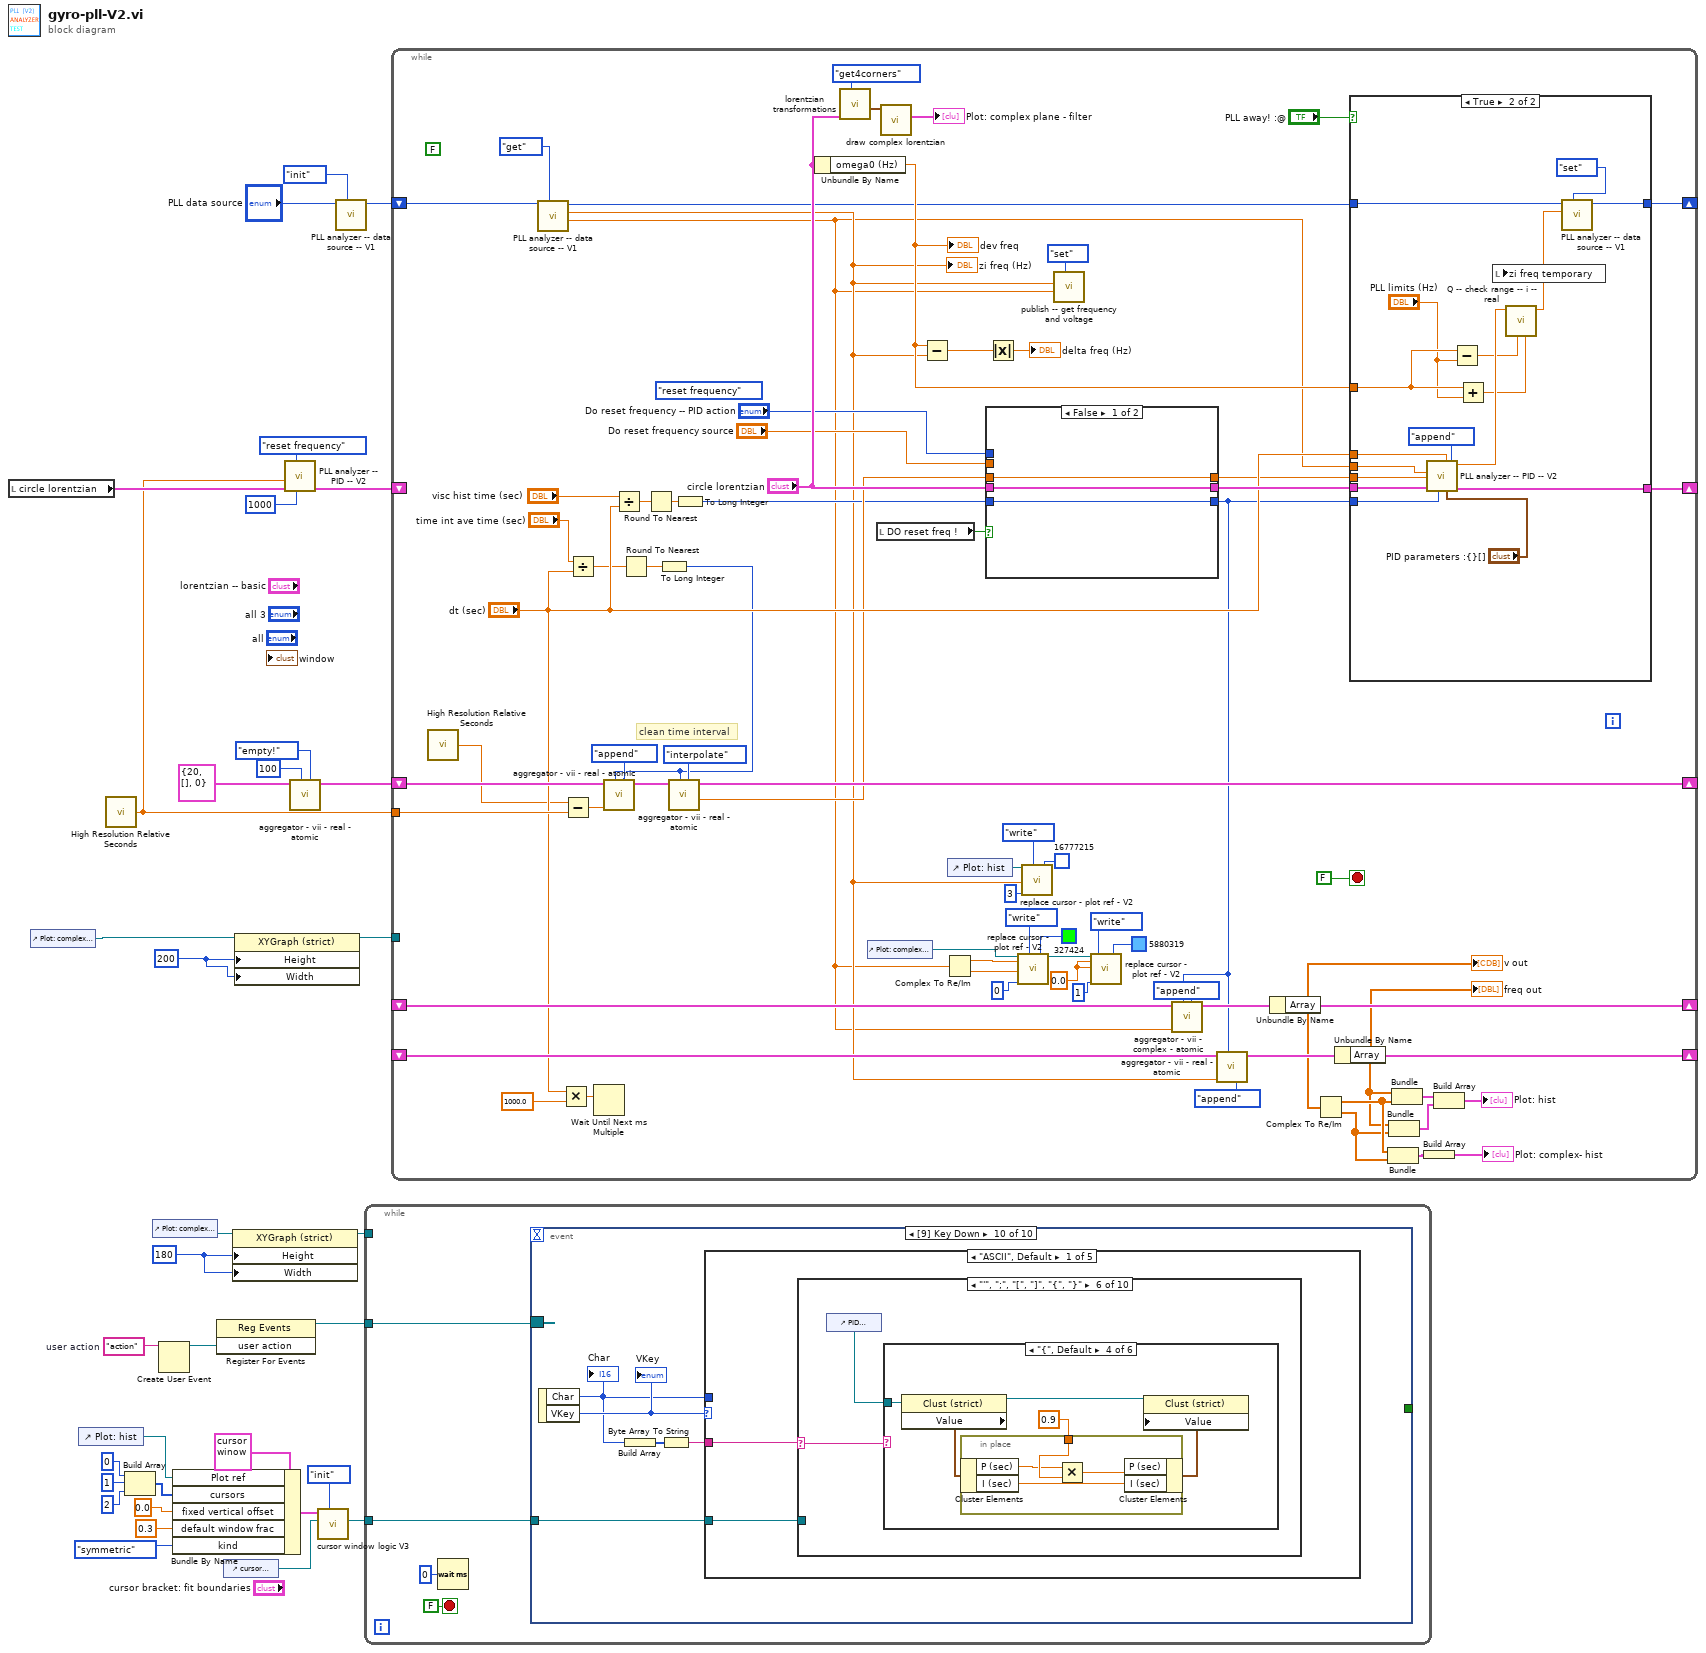
[diagram p0: block diagram]
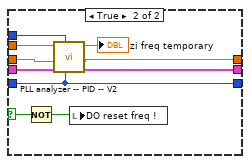
[diagram p3: hidden frame]
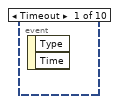
[diagram p4: hidden frame]
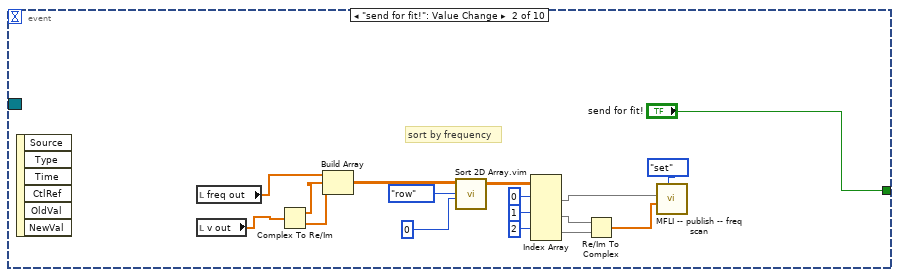
[diagram p5: hidden frame]
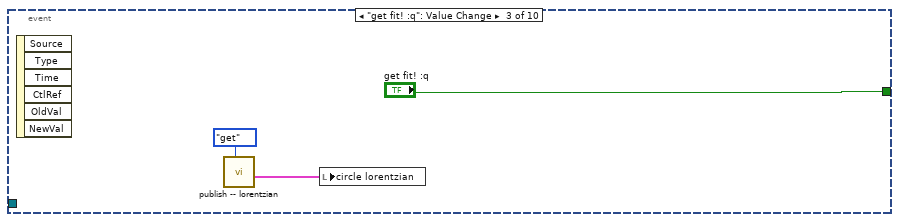
[diagram p6: hidden frame]
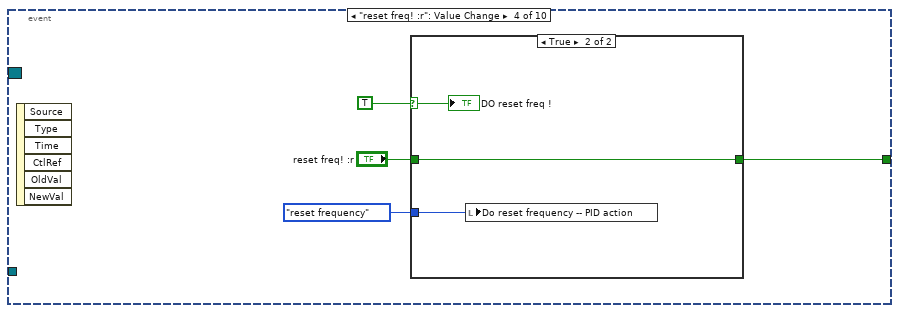
[diagram p7: hidden frame]
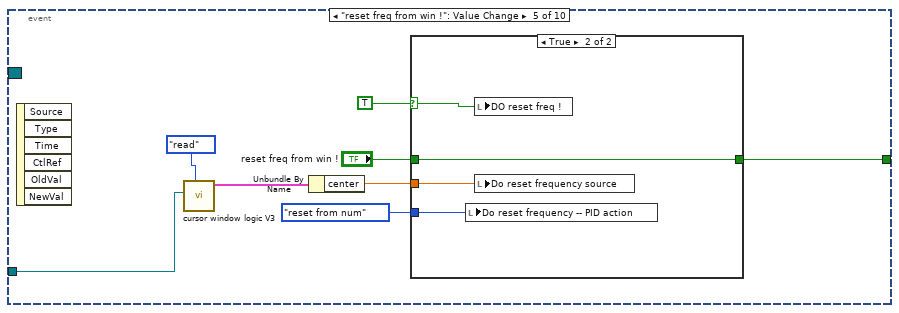
[diagram p9: hidden frame]
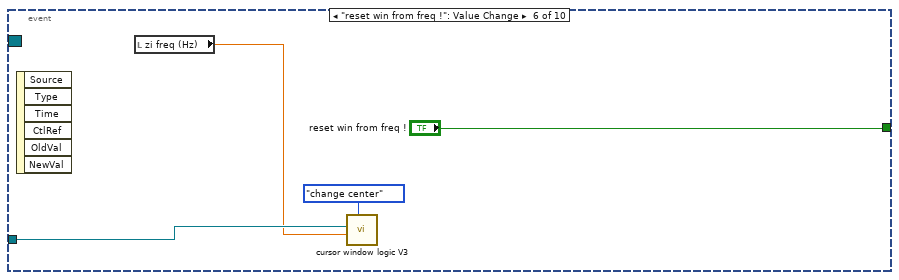
[diagram p11: hidden frame]
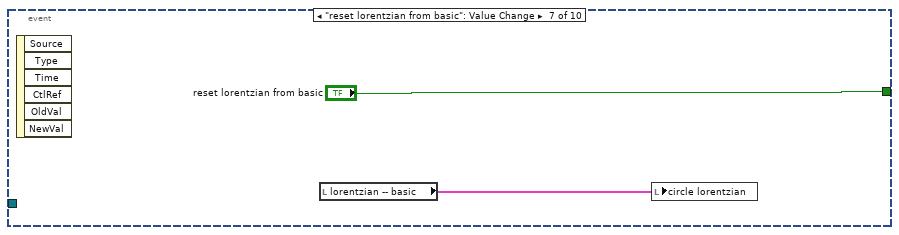
[diagram p12: hidden frame]
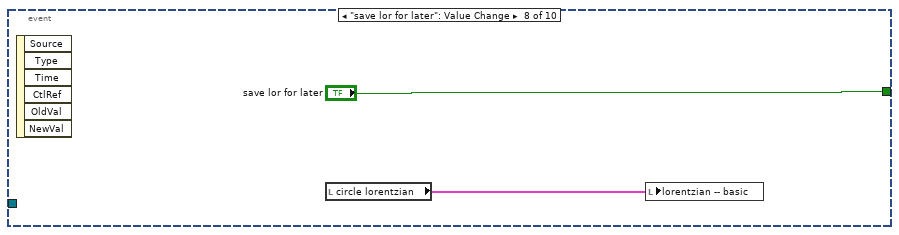
[diagram p13: hidden frame]
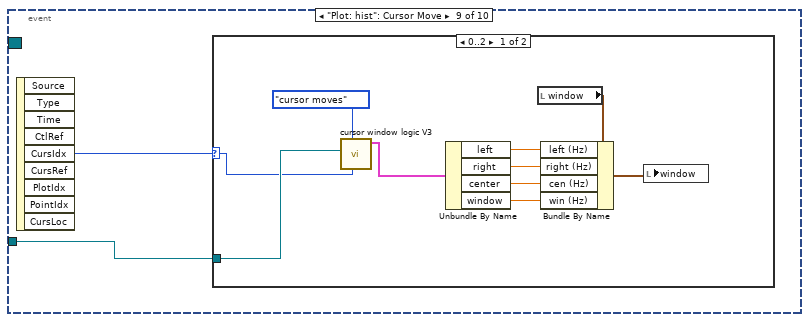
[diagram p14: hidden frame]
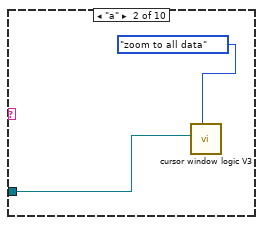
[diagram p17: hidden frame]
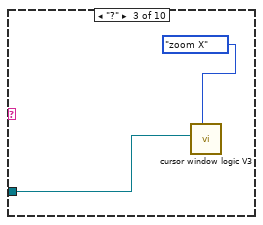
[diagram p18: hidden frame]
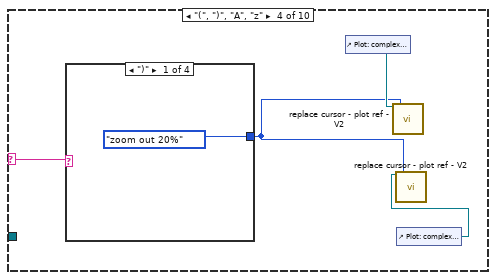
[diagram p19: hidden frame]
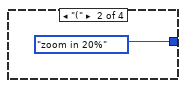
[diagram p20: hidden frame]
diagram:
  w8 = u32 180 ("Plot Area:Size:Height")
  w10 = u32 200 ("Plot Area:Size:Height")
  w31 = "action"  # user action
  n1 = local read "circle lorentzian"() -> (w15:T2)
  n2 = control-ref of="Plot: complex plane - filter"() -> (w11:refnum<vi>)
  n3 = control-ref of="Plot: hist"() -> (w7:refnum<vi>)
  n4 = call <vilib>:"High Resolution Relative Seconds.vi"() -> ("relative seconds"=w1:dbl)
  n5 = Build Array(0, 1, 2) -> (w19:i32[])
  n6 = control-ref of="Plot: complex- hist"() -> (w5:refnum<vi>)
  n7 = Create User Event(user event datatype=w31) -> (user event=w32:refnum<user-event>)  [unwired: 1 in, 1 out]
  n8 = Bundle By Name(cluster=T5 {"left"=0.0, "right "=0.0, "center"=0.0, "window"=0.0, "cursors"=[], "relative"=0, "absolute"=0, "fixed vertical offset"=0.0, "vertical offset"=0.0, "skew"=0.0, "default window frac"=0.0, "kind"=enum."symmetric", "skew.left"=0.0, "skew.right"=0.0, "Plot ref"=refnum, "wing order"=enum."forw"} ("cursor bracket: All, data window"), "Plot ref"=w7, "cursors"=w19, "fixed vertical offset"=0.0, "default window frac"=0.3 ("fixed vertical offset"), "kind"=enum16{"symmetric", "skewed", "fancy"}."symmetric") -> (w27:T5)
  n9 = register-events(w32) -> (reference out=w30:refnum<event-registration>)  [unwired: 2 in, 1 out]
  n10 = control-ref of="cursor bracket: fit boundaries"() -> (w29:refnum<vi>)
  n11 = property class="XYGraph (strict)"(reference=w5, "Height"=w8, "Width"=w8) -> (reference out=w6:refnum<vi>)  [unwired: 1 in, 1 out]
  n12 = property class="XYGraph (strict)"(reference=w11, "Height"=w10, "Width"=w10) -> (reference out=w9:refnum<vi>)  [unwired: 1 in, 1 out]
  n13 = call "PLL analyzer -- PID -- V2.vi"("requested size"=1000, "PID action"=PID_action."reset frequency", "lorentzian IN"=w15, "time in (sec)"=w1) -> ("lorentzian  OUT"=w14:T2)  [unwired: 5 in, 2 out]
  n14 = call "aggregator - vii - real - atomic.vi"("aggregator action"=agregator_--_action."empty!", "requested size"=100, "state IN"=T10 {"requested size"=20, "Array"=[], "actual number of elements"=0}) -> ("state OUT"=w18:T10)  [unwired: 5 in, 3 out]
  n15 = call "cursor window logic V3.vi"("cursor window action"=cursor_window_action."init", "cursor window in"=w29, "cursor window init"=w27) -> ("cursor window out"=w33:refnum<vi>)  [unwired: 7 in, 1 out]
  n16 = call "PLL analyzer -- data source -- V1.vi"("data source action"=data_source_action."init", "PLL data source"="PLL data source") -> ("PLL data source OUT"=w2:T4)  [unwired: 7 in, 2 out]
  n17 = while {
    tunnel: w30 -> [w38]
    tunnel: w33 -> [w36]
    tunnel: w6 -> [_]
    stop <- FALSE stop-if-true
    n18 = Wait (ms)(milliseconds to wait=u32 0) -> ()  [unwired: 1 out]
    n19 = event shown="[9] Key Down" {
      selector: w38 -> [_ _ _ _ _ _ _ _ _ _]
      dyn-events: _ -> [_ _ _ _ _ _ _ _ _ _]
      timeout: _ -> [_ _ _ _ _ _ _ _ _ _]
      tunnel: w36 -> [_ _ _ _ w69 w82 _ _ w89 w100]
      tunnel: [_ "send for fit!" "get fit! :q" w61 w73 "reset win from freq !" "reset lorentzian from basic" "save lor for later" _ _] -> _
      event Timeout {
        n20 = event-data() -> ()  [unwired: 1 in, 2 out]
      }
      event "send for fit!": Value Change {
        # "sort by frequency"
        n21 = event-data() -> ()  [unwired: 1 in, 6 out]
        n22 = local read "freq out"() -> (w48:dbl[])
        n23 = local read "v out"() -> (w46:cdb[])
        n24 = Complex To Re/Im(x + iy=w46) -> (x=w45:dbl[], y=w44:dbl[])
        n25 = Build Array(w48, w45, w44) -> (w47:dbl[][])
        n26 = call "Sort 2D Array.vim"("index"=0, "dimension to index (column)"=enum16{"column", "row"}."row", "2D array"=w47) -> ("sorted 2D array"=w53:dbl[][])  [unwired: 7 in, 1 out]
        n27 = Index Array(array=w53, index (row) #1=0 ("index (row)"), index (row) #2=1 ("index (row)"), index (row) #3=2 ("index (row)")) -> (element #1=w42:dbl[], element #2=w41:dbl[], element #3=w40:dbl[])  [unwired: 3 in]
        n28 = Re/Im To Complex(1:w40, 2:w41) -> (0:w39:cdb[])
        n29 = call "MFLI -- publish -- freq scan.vi"("publisher action"=publisher_action."set", "Voltage IN (V)"=w39, "Freq IN (Hz)"=w42) -> ()  [unwired: 7 in, 2 out]
      }
      event "get fit! :q": Value Change {
        n30 = event-data() -> ()  [unwired: 1 in, 6 out]
        n31 = call "publish -- lorentzian.vi"("publisher action"=publisher_action."get") -> ("lorentzian OUT"=w56:T2)  [unwired: 10 in]
        n32 = local write "circle lorentzian"(w56) -> ()
      }
      event "reset freq! :r": Value Change {
        n33 = event-data() -> ()  [unwired: 1 in, 6 out]
        n34 = case shown="True" TRUE ("DO reset freq !") {
          selector: TRUE ("DO reset freq !") -> [_ w66]
          tunnel: [w63 w65] -> w61
          tunnel: "reset freq! :r" -> [w63 w65]
          tunnel: PID_action."reset frequency" ("PID action") -> [_ w64]
          frame False {
          }
          frame True {
            n35 = local write "Do reset frequency -- PID action"(w64) -> ()
            "DO reset freq !" <- w66
          }
        }
      }
      event "reset freq from win !": Value Change {
        n36 = event-data() -> ()  [unwired: 1 in, 6 out]
        n37 = call "cursor window logic V3.vi"("cursor window action"=cursor_window_action."read", "cursor window in"=w69) -> ("cursor window out"=w68:T5)  [unwired: 8 in, 1 out]
        n38 = Unbundle By Name(w68) -> ("center"=w67:dbl)
        n39 = case shown="True" TRUE ("DO reset freq !") {
          selector: TRUE ("DO reset freq !") -> [_ w77]
          tunnel: [w75 w79] -> w73
          tunnel: "reset freq from win !" -> [w75 w79]
          tunnel: PID_action."reset from num" ("PID action") -> [_ w78]
          tunnel: w67 -> [_ w76]
          frame False {
          }
          frame True {
            n40 = local write "Do reset frequency -- PID action"(w78) -> ()
            n41 = local write "DO reset freq !"(w77) -> ()
            n42 = local write "Do reset frequency source"(w76) -> ()
          }
        }
      }
      event "reset win from freq !": Value Change {
        n43 = event-data() -> ()  [unwired: 1 in, 6 out]
        n44 = local read "zi freq (Hz)"() -> (w81:dbl)
        n45 = call "cursor window logic V3.vi"("cursor window action"=cursor_window_action."change center", "center"=w81, "cursor window in"=w82) -> ()  [unwired: 7 in, 2 out]
      }
      event "reset lorentzian from basic": Value Change {
        n46 = event-data() -> ()  [unwired: 1 in, 6 out]
        n47 = local read "lorentzian -- basic"() -> (w84:T2)
        n48 = local write "circle lorentzian"(w84) -> ()
      }
      event "save lor for later": Value Change {
        n49 = event-data() -> ()  [unwired: 1 in, 6 out]
        n50 = local read "circle lorentzian"() -> (w86:T2)
        n51 = local write "lorentzian -- basic"(w86) -> ()
      }
      event "Plot: hist": Cursor Move {
        n52 = event-data() -> ("CursIdx"=w88:i32)  [unwired: 1 in, 8 out]
        n53 = case shown="0..2" w88 {
          selector: w88 -> [w97 _]
          tunnel: w89 -> [w99 _]
          frame 0..2 {
            n54 = call "cursor window logic V3.vi"("CursIdx"=w97, "cursor window action"=cursor_window_action."cursor moves", "cursor window in"=w99) -> ("cursor window out"=w96:T5)  [unwired: 7 in, 1 out]
            n55 = Unbundle By Name(w96) -> ("left"=w94:dbl, "right"=w93:dbl, "center"=w92:dbl, "window"=w91:dbl)
            n56 = local read "window"() -> (w95:T8)
            n57 = Bundle By Name(cluster=w95, "left (Hz)"=w94, "right (Hz)"=w93, "cen (Hz)"=w92, "win (Hz)"=w91) -> (w90:T8)
            n58 = local write "window"(w90) -> ()
          }
          frame 3, Default {
          }
        }
      }
      event Key Down {
        n59 = event-data() -> ("Char"=w102:i16, "VKey"=w104:T6)  [unwired: 1 in]
        "Char" <- w102
        "VKey" <- w104
        n60 = Build Array(w102) -> (w103:i16[])
        n61 = Byte Array To String(unsigned byte array=w103) -> (string=w101:string)
        n62 = case shown="\"ASCII\", Default" w104 {
          selector: w104 -> [_ _ _ _ w201]
          tunnel: w102 -> [_ _ _ _ _]
          tunnel: w101 -> [w106 _ _ _ _]
          tunnel: w100 -> [w105 _ _ _ w199]
          frame "ASCII", Default {
            n63 = case shown="\"'\", \";\", \"[\", \"]\", \"{\", \"}\"" w106 {
              selector: w106 -> [_ _ _ w111 _ w122 _ w182 _ _]
              tunnel: w105 -> [_ w107 w109 _ _ _ _ w183 w188 _]
              frame "0", Default {
              }
              frame "a" {
                n64 = call "cursor window logic V3.vi"("cursor window action"=cursor_window_action."zoom to all data", "cursor window in"=w107) -> ()  [unwired: 8 in, 2 out]
              }
              frame "?" {
                n65 = call "cursor window logic V3.vi"("cursor window action"=cursor_window_action."zoom X", "cursor window in"=w109) -> ()  [unwired: 8 in, 2 out]
              }
              frame "(", ")", "A", "z" {
                n66 = case shown="\")\"" w111 {
                  tunnel: [cursor_action."zoom out 20%" ("cursor action") cursor_action."zoom in 20%" ("cursor action") cursor_action."smart zoom out" ("cursor action") cursor_action."zoom to aspect ratio 1" ("cursor action")] -> w113
                  frame ")" {
                  }
                  frame "(" {
                  }
                  frame "A" {
                  }
                  frame "z", Default {
                  }
                }
                n67 = control-ref of="Plot: complex plane - filter"() -> (w114:refnum<vi>)
                n68 = call "replace cursor - plot ref - V2.vi"("Plot ref in"=w114, "cursor action"=w113) -> ()  [unwired: 15 in, 3 out]
                n69 = control-ref of="Plot: complex- hist"() -> (w112:refnum<vi>)
                n70 = call "replace cursor - plot ref - V2.vi"("Plot ref in"=w112, "cursor action"=w113) -> ()  [unwired: 15 in, 3 out]
              }
              frame "r" {
                n71 = local write "DO reset freq !"(TRUE ("DO reset freq !")) -> ()
                n72 = local write "Do reset frequency -- PID action"(PID_action."reset frequency" ("PID action")) -> ()
              }
              frame "'", ";", "[", "]", "{", "}" {
                n73 = control-ref of="PID parameters :{}[];'"() -> (w121:refnum<vi>)
                n74 = case shown="\"{\", Default" w122 {
                  tunnel: w121 -> [w127 w136 w145 w154 w163 w173]
                  frame "[" {
                    n75 = property class="Clust (strict)"(reference=w127) -> (reference out=w126:refnum<vi>, "Value"=w125:T1)  [unwired: 1 in, 1 out]
                    n76 = in-place {
                      in-place-border: 0.9 -> [w130]
                      n77 = in-place-cluster #1(w125) -> ("P (sec)"=w128:dbl, "I (sec)"=w131:dbl)
                      n78 = Multiply(x=w131, y=w130) -> (x*y=w129:dbl)
                      n79 = in-place-cluster #1("P (sec)"=w128, "I (sec)"=w129) -> (w124:T1)
                    }
                    n80 = property class="Clust (strict)"(reference=w126, "Value"=w124) -> ()  [unwired: 1 in, 2 out]
                  }
                  frame "]" {
                    n81 = property class="Clust (strict)"(reference=w136) -> (reference out=w135:refnum<vi>, "Value"=w134:T1)  [unwired: 1 in, 1 out]
                    n82 = in-place {
                      in-place-border: 1.1 -> [w139]
                      n83 = in-place-cluster #2(w134) -> ("P (sec)"=w137:dbl, "I (sec)"=w140:dbl)
                      n84 = Multiply(x=w140, y=w139) -> (x*y=w138:dbl)
                      n85 = in-place-cluster #2("P (sec)"=w137, "I (sec)"=w138) -> (w133:T1)
                    }
                    n86 = property class="Clust (strict)"(reference=w135, "Value"=w133) -> ()  [unwired: 1 in, 2 out]
                  }
                  frame "}" {
                    n87 = property class="Clust (strict)"(reference=w145) -> (reference out=w144:refnum<vi>, "Value"=w143:T1)  [unwired: 1 in, 1 out]
                    n88 = in-place {
                      in-place-border: 1.1 -> [w149]
                      n89 = in-place-cluster #3(w143) -> ("P (sec)"=w148:dbl, "I (sec)"=w146:dbl)
                      n90 = Multiply(x=w148, y=w149) -> (x*y=w147:dbl)
                      n91 = in-place-cluster #3("P (sec)"=w147, "I (sec)"=w146) -> (w142:T1)
                    }
                    n92 = property class="Clust (strict)"(reference=w144, "Value"=w142) -> ()  [unwired: 1 in, 2 out]
                  }
                  frame "{", Default {
                    n93 = property class="Clust (strict)"(reference=w154) -> (reference out=w153:refnum<vi>, "Value"=w152:T1)  [unwired: 1 in, 1 out]
                    n94 = in-place {
                      in-place-border: 0.9 -> [w158]
                      n95 = in-place-cluster #4(w152) -> ("P (sec)"=w157:dbl, "I (sec)"=w155:dbl)
                      n96 = Multiply(x=w157, y=w158) -> (x*y=w156:dbl)
                      n97 = in-place-cluster #4("P (sec)"=w156, "I (sec)"=w155) -> (w151:T1)
                    }
                    n98 = property class="Clust (strict)"(reference=w153, "Value"=w151) -> ()  [unwired: 1 in, 2 out]
                  }
                  frame "'" {
                    n99 = property class="Clust (strict)"(reference=w163) -> (reference out=w162:refnum<vi>, "Value"=w161:T1)  [unwired: 1 in, 1 out]
                    n100 = in-place {
                      in-place-border: 1.1 -> [w164]
                      n101 = in-place-cluster #5(w161) -> ("P (sec)"=w168:dbl, "I (sec)"=w166:dbl)
                      n102 = Multiply(x=w168, y=w164) -> (x*y=w167:dbl)
                      n103 = Multiply(x=w166, y=w164) -> (x*y=w165:dbl)
                      n104 = in-place-cluster #5("P (sec)"=w167, "I (sec)"=w165) -> (w160:T1)
                    }
                    n105 = property class="Clust (strict)"(reference=w162, "Value"=w160) -> ()  [unwired: 1 in, 2 out]
                  }
                  frame ";" {
                    n106 = property class="Clust (strict)"(reference=w173) -> (reference out=w172:refnum<vi>, "Value"=w171:T1)  [unwired: 1 in, 1 out]
                    n107 = in-place {
                      in-place-border: 0.9 -> [w174]
                      n108 = in-place-cluster #6(w171) -> ("P (sec)"=w178:dbl, "I (sec)"=w176:dbl)
                      n109 = Multiply(x=w178, y=w174) -> (x*y=w177:dbl)
                      n110 = Multiply(x=w176, y=w174) -> (x*y=w175:dbl)
                      n111 = in-place-cluster #6("P (sec)"=w177, "I (sec)"=w175) -> (w170:T1)
                    }
                    n112 = property class="Clust (strict)"(reference=w172, "Value"=w170) -> ()  [unwired: 1 in, 2 out]
                  }
                }
              }
              frame "@" {
                n113 = local read "PLL away! :@"() -> (w180:bool)
                n114 = Not(x=w180) -> (.not. x?=w179:bool)
                n115 = local write "PLL away! :@"(w179) -> ()
              }
              frame "+", "-", "<", ">" {
                # "?"
                n116 = case shown="\"+\", Default" w182 {
                  tunnel: [cursor_window_action."slide right" ("cursor window action") cursor_window_action."slide left" ("cursor window action") cursor_window_action."zoom in" ("cursor window action") cursor_window_action."zoom out" ("cursor window action")] -> w181
                  frame ">" {
                  }
                  frame "<" {
                  }
                  frame "+", Default {
                  }
                  frame "-" {
                  }
                }
                n117 = call "cursor window logic V3.vi"("cursor window action"=w181, "cursor window in"=w183) -> ()  [unwired: 8 in, 2 out]
              }
              frame "c" {
                n118 = call "cursor window logic V3.vi"("cursor window action"=cursor_window_action."check", "cursor window in"=w188) -> ()  [unwired: 8 in, 2 out]
              }
              frame "q" {
                n119 = call "publish -- lorentzian.vi"("publisher action"=publisher_action."get") -> ("lorentzian OUT"=w190:T2)  [unwired: 10 in]
                n120 = local write "circle lorentzian"(w190) -> ()
              }
            }
          }
          frame "Escape" {
          }
          frame "PageUp" {
          }
          frame "PageDown" {
          }
          frame "Up".."Right" {
            n121 = case shown="\"Left\"" w201 {
              tunnel: [cursor_window_action."move right" ("cursor window action") cursor_window_action."move left" ("cursor window action") cursor_window_action."broaden" ("cursor window action") cursor_window_action."shrink" ("cursor window action")] -> w200
              frame "Right", Default {
              }
              frame "Left" {
              }
              frame "Up" {
              }
              frame "Down" {
              }
            }
            n122 = call "cursor window logic V3.vi"("cursor window action"=w200, "cursor window in"=w199) -> ("cursor window out"=w192:T5)  [unwired: 8 in, 1 out]
            n123 = Unbundle By Name(w192) -> ("left"=w194:dbl, "right"=w195:dbl, "center"=w196:dbl, "window"=w197:dbl)
            n124 = local read "window"() -> (w193:T8)
            n125 = Bundle By Name(cluster=w193, "left (Hz)"=w194, "right (Hz)"=w195, "cen (Hz)"=w196, "win (Hz)"=w197) -> (w198:T8)
            n126 = local write "window"(w198) -> ()
          }
        }
      }
    }
  }
  n127 = while {
    tunnel: w1 -> [w278]
    shift-right: [w269] -> _
    shift-left: w14 -> [_]
    shift-right: [w259] -> _
    shift-left: _ -> [w265]
    shift-right: [w260] -> _
    shift-left: _ -> [w262]
    shift-right: [w248] -> _
    shift-left: w18 -> [w251]
    shift-right: [w239] -> _
    shift-left: w2 -> [w226]
    tunnel: w9 -> [_]
    stop <- FALSE stop-if-true
    w216 = 0.0 ("new X")
    (unwired) PID_action."reset frequency" ("PID action")
    (unwired) FALSE
    # "clean time interval"
    n128 = call <vilib>:"High Resolution Relative Seconds.vi"() -> ("relative seconds"=w229:dbl)
    n129 = call "PLL analyzer -- data source -- V1.vi"("data source action"=data_source_action."get", "PLL data source"=w226) -> ("z out (V)"=w207:cdb, "Freq out (Hz)"=w208:dbl, "PLL data source OUT"=w228:T4)  [unwired: 7 in]
    "zi freq (Hz)" <- w208
    n130 = Multiply(x="dt (sec)", y=1000.0) -> (x*y=w244:dbl)
    n131 = Subtract(x=w229, y=w278) -> (x-y=w250:dbl)
    n132 = Divide(x="time int ave time (sec)", y="dt (sec)") -> (x/y=w212:dbl)
    n133 = Wait Until Next ms Multiple(millisecond multiple=w244) -> ()  [unwired: 1 out]
    n134 = Divide(x="visc hist time (sec)", y="dt (sec)") -> (x/y=w215:dbl)
    n135 = Round To Nearest(number=w212) -> (nearest integer value=w211:dbl)
    n136 = Round To Nearest(number=w215) -> (nearest integer value=w214:dbl)
    n137 = To Long Integer(number=w211) -> (32bit integer=w210:i32)
    n138 = call "aggregator - vii - real - atomic.vi"("aggregator action"=agregator_--_action."append", "requested size"=w210, "number"=w250, "state IN"=w251) -> ("state OUT"=w249:T10)  [unwired: 4 in, 3 out]
    n139 = call "aggregator - vii - real - atomic.vi"("aggregator action"=agregator_--_action."interpolate", "requested size"=w210, "state IN"=w249) -> ("interp average"=w223:dbl, "state OUT"=w248:T10)  [unwired: 5 in, 2 out]
    n140 = To Long Integer(number=w214) -> (32bit integer=w213:i32)
    n141 = Unbundle By Name("circle lorentzian") -> ("omega0 (Hz)"=w235:dbl)
    "dev freq" <- w235
    n142 = call "lorentzian transformations.vi"("4 corner circle transformation"=four-corner_circle_transformation."get4corners", "lorentzian in"="circle lorentzian") -> ("4corners our"=w276:T3)  [unwired: 7 in, 2 out]
    n143 = control-ref of="Plot: complex plane - filter"() -> (w224:refnum<vi>)
    n144 = local read "DO reset freq !"() -> (w243:bool)
    n145 = call "draw complex lorentzian.vi"("4 corners"=w276) -> ("fancy circles"=→"Plot: complex plane - filter":cluster{dbl[], dbl[]}[])  [unwired: 10 in]
    n146 = Subtract(x=w235, y=w208) -> (x-y=w257:dbl)
    n147 = Complex To Re/Im(x + iy=w207) -> (x=w271:dbl, y=w270:dbl)
    n148 = control-ref of="Plot: hist"() -> (w230:refnum<vi>)
    n149 = case shown="False" w243 {
      selector: w243 -> [_ w308]
      tunnel: "circle lorentzian" -> [w300 w310]
      tunnel: [w300 w309] -> w241
      tunnel: w213 -> [w299 w305]
      tunnel: [w299 w305] -> w225
      tunnel: w223 -> [w298 w304]
      tunnel: "Do reset frequency -- PID action" -> [_ w303]
      tunnel: "Do reset frequency source" -> [_ w302]
      tunnel: [w298 w301] -> w206
      frame False {
      }
      frame True {
        n150 = Not(x=w308) -> (.not. x?=w307:bool)
        n151 = call "PLL analyzer -- PID -- V2.vi"("requested size"=w305, "PID action"=w303, "lorentzian IN"=w310, "time in (sec)"=w304, "frequency IN (Hz)"=w302) -> ("lorentzian  OUT"=w309:T2, "time out (sec)"=w301:dbl, "frequency OUT (Hz)"=→"zi freq temporary":dbl)  [unwired: 4 in]
        n152 = local write "DO reset freq !"(w307) -> ()
      }
    }
    n153 = Absolute Value(x=w257) -> (abs(x)=→"delta freq (Hz)":dbl)
    n154 = call "replace cursor - plot ref - V2.vi"("Plot ref in"=w224, "new X"=w271, "new  Y"=w270, "cursor index"=0, "cursor action"=cursor_action."write", "Color Box"=u32 327424) -> ("Plot ref out"=w220:refnum<vi>)  [unwired: 11 in, 2 out]
    n155 = call "replace cursor - plot ref - V2.vi"("Plot ref in"=w230, "new  Y"=w208, "cursor index"=3, "cursor action"=cursor_action."write", "Color Box"=u32 16777215) -> ()  [unwired: 12 in, 3 out]
    n156 = call "publish -- get frequency and voltage.vi"("publisher action"=publisher_action."set", "Voltage IN (V)"=w207, "freq IN (Hz)"=w208) -> ()  [unwired: 7 in, 2 out]
    n157 = call "replace cursor - plot ref - V2.vi"("Plot ref in"=w220, "new X"=w216, "new  Y"=w216, "cursor index"=1, "cursor action"=cursor_action."write", "Color Box"=u32 5880319) -> ()  [unwired: 11 in, 3 out]
    n158 = call "aggregator - vii - complex - atomic.vi"("aggregator action"=agregator_--_action."append", "requested size"=w225, "number"=w207, "state IN"=w265) -> ("state OUT"=w259:T16)  [unwired: 4 in, 3 out]
    n159 = call "aggregator - vii - real - atomic.vi"("aggregator action"=agregator_--_action."append", "requested size"=w225, "number"=w208, "state IN"=w262) -> ("state OUT"=w260:T10)  [unwired: 4 in, 3 out]
    n160 = Unbundle By Name(w259) -> ("Array"=w258:cdb[])
    "v out" <- w258
    n161 = Complex To Re/Im(x + iy=w258) -> (x=w255:dbl[], y=w254:dbl[])
    n162 = Unbundle By Name(w260) -> ("Array"=w245:dbl[])
    "freq out" <- w245
    n163 = case shown="True" "PLL away! :@" {
      tunnel: [w280 w297] -> w269
      tunnel: w225 -> [_ w295]
      tunnel: w207 -> [_ w283]
      tunnel: w206 -> [_ w282]
      tunnel: w241 -> [w280 w294]
      tunnel: [w279 w286] -> w239
      tunnel: w228 -> [w279 w284]
      tunnel: w235 -> [_ w291]
      tunnel: "dt (sec)" -> [_ w288]
      frame False {
      }
      frame True {
        n164 = call "PLL analyzer -- PID -- V2.vi"("PID parameters"="PID parameters :{}[]", "dt (sec)"=w288, "requested size"=w295, "PID action"=PID_action."append", "lorentzian IN"=w294, "time in (sec)"=w282, "voltage IN (V)"=w283) -> ("lorentzian  OUT"=w297:T2, "frequency OUT (Hz)"=w293:dbl)  [unwired: 2 in, 1 out]
        n165 = Subtract(x=w291, y="PLL limits (Hz)") -> (x-y=w289:dbl)
        n166 = Add(x=w291, y="PLL limits (Hz)") -> (x+y=w292:dbl)
        n167 = call "Q -- check range -- i -- real.vi"("upper"=w292, "lower"=w289, "number"=w293) -> ("number in range"=w281:dbl)  [unwired: 6 in, 2 out]
        n168 = local write "zi freq temporary"(w281) -> ()
        n169 = call "PLL analyzer -- data source -- V1.vi"("data source action"=data_source_action."set", "Freq in (Hz)"=w281, "PLL data source"=w284) -> ("PLL data source OUT"=w286:T4)  [unwired: 6 in, 2 out]
      }
    }
    n170 = Bundle(w255, w254) -> (w256:cluster{dbl[], dbl[]})  [unwired: 1 in]
    n171 = Bundle("Array"=w245, w254) -> (w267:cluster{"Array":dbl[], dbl[]})  [unwired: 1 in]
    n172 = Bundle("Array"=w245, w255) -> (w268:cluster{"Array":dbl[], dbl[]})  [unwired: 1 in]
    n173 = Build Array(w256) -> (→"Plot: complex- hist":cluster{dbl[], dbl[]}[])
    n174 = Build Array(w268, w267) -> (→"Plot: hist":cluster{"Array":dbl[], dbl[]}[])
  }
